vi "Set Value U64.vi"(0 "Session Handle in":T1, 1 "Create If Missing? (T)":bool=TRUE, 5 "Lookup String":string, 9 "Value":u64, 11 "error in (no error)":errorcluster) -> (4 "Session Handle out":T1, 15 "error out":errorcluster)   [LabVIEW 2019, in "HTS.lvlib" / "VariableContainer.lvclass"]
uses:
  VariableContainer.lvclass
  <vilib>/addons/TestStand/_TSUtility.llb/TestStand API Numeric Constants.ctl
  Typedefs/Session Handle.ctl
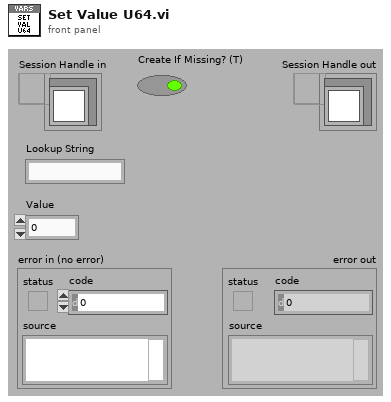
[diagram p1: front panel]
types:
  T1 = typedef "HTS.lvlib/VariableContainer.lvclass/Session Handle.ctl" = refnum<data-value>
  T2 = typedef "TestStand API Numeric Constants.ctl" = enum16{"APILocation_ActiveXModule_ActiveXReferenceExpr", "APILocation_ActiveXModule_FilePath", "APILocation_ActiveXModule_RemoteHost", "APILocation_ActiveXParameter_ValueExpr", "APILocation_AdditionalResult_Condition", "APILocation_AdditionalResult_Name", "APILocation_AdditionalResult_ValueToLog", "APILocation_CommonCModule_ModulePath", "APILocation_CommonCModule_ProjectFilePath", "APILocation_CommonCModule_SourceFilePath", "APILocation_CommonCModule_WorkspaceFilePath", "APILocation_CommonCParameter_StringBufferSizeExpr", "APILocation_CommonCParameter_ValueExpr", "APILocation_DllParameter_ImaginaryPartValueExpr", "APILocation_DotNetModule_GetAssembly", "APILocation_DotNetModule_ProjectFilePath", "APILocation_DotNetModule_SolutionFilePath", "APILocation_DotNetModule_SourceFilePath", "APILocation_DotNetParameter_ParameterName", "APILocation_DotNetParameter_ValueExpr", "APILocation_HTBasicModule_SubroutineFilePath", "APILocation_LabVIEWModule_CallName", "APILocation_LabVIEWModule_ClassPath", "APILocation_LabVIEWModule_GetVIAbsolutePath", "APILocation_LabVIEWModule_NodeLibraryName", "APILocation_LabVIEWModule_OverrideBinaryClassPath", "APILocation_LabVIEWModule_OverrideBinaryProjectPath", "APILocation_LabVIEWModule_OverrideBinaryVIPath", "APILocation_LabVIEWModule_OverrideSourceClassPath", "APILocation_LabVIEWModule_OverrideSourceProjectPath", "APILocation_LabVIEWModule_OverrideSourceVIPath", "APILocation_LabVIEWModule_ProjectPath", "APILocation_LabVIEWModule_RemoteConnectionTimeout", "APILocation_LabVIEWModule_RemoteHost", "APILocation_LabVIEWModule_RemotePortNumber", "APILocation_LabVIEWModule_VIPath", "APILocation_LabVIEWModule_VIType", "APILocation_LabVIEWNXGModule_GllPath", "APILocation_LabVIEWNXGModule_ModuleQualifiedName", "APILocation_LabVIEWNXGModule_ProjectPath", "APILocation_LabVIEWNXGModule_QualifiedName", "APILocation_LabVIEWNXGParameter_ParameterLabel", "APILocation_LabVIEWNXGParameter_Type", "APILocation_LabVIEWNXGParameter_ValueExpression", "APILocation_LabVIEWParameterElement_ElementCaption", "APILocation_LabVIEWParameterElement_ValueExpr", "APILocation_LabVIEWParameter_ParameterCaption", "APILocation_LabVIEWParameter_ValueExpr", "APILocation_None", "APILocation_PythonModule_ClassInstanceLocationExpr", "APILocation_PythonModule_ClassName", "APILocation_PythonModule_FunctionOrAttributeName", "APILocation_PythonModule_InterpreterReferenceExpr", "APILocation_PythonModule_ModulePath", "APILocation_PythonModule_PythonVersion", "APILocation_PythonModule_PythonVirtualEnvironmentPath", "APILocation_PythonParameter_ValueExpr", "APILocation_SequenceCallModule_CustomCPUAffinityForNewThread", "APILocation_SequenceCallModule_NewExecutionBreakOnEntryExpr", "APILocation_SequenceCallModule_NewExecutionModelPath", "APILocation_SequenceCallModule_NewExecutionTypeMaskExpr", "APILocation_SequenceCallModule_RemoteHost", "APILocation_SequenceCallModule_SequenceFilePath", "APILocation_SequenceCallModule_SequenceName", "APILocation_SequenceCallModule_StoreActiveXReferenceExpr", "APILocation_SequenceCallParameter_ValueExpr", "APILocation_SequenceFile_ModelPath", "APILocation_Sequence_DisableResults", "APILocation_StepType_BatchSyncOption", "APILocation_StepType_CustomActionExpression", "APILocation_StepType_CustomFalseAction", "APILocation_StepType_CustomFalseActionTargetByExpr", "APILocation_StepType_CustomTrueAction", "APILocation_StepType_CustomTrueActionTargetByExpr", "APILocation_StepType_DefaultNameExpr", "APILocation_StepType_DescriptionExpr", "APILocation_StepType_EvalPrecondForInteractiveExecution", "APILocation_StepType_FailAction", "APILocation_StepType_FailActionTargetByExpr", "APILocation_StepType_IconName", "APILocation_StepType_IgnoreRTE", "APILocation_StepType_LoopIncExpression", "APILocation_StepType_LoopInitExpression", "APILocation_StepType_LoopStatusExpression", "APILocation_StepType_LoopType", "APILocation_StepType_LoopWhileExpression", "APILocation_StepType_MenuItemNameExpr", "APILocation_StepType_ModuleLoadOption", "APILocation_StepType_ModuleUnloadOption", "APILocation_StepType_MutexNameOrRefExpr", "APILocation_StepType_PassAction", "APILocation_StepType_PassActionTargetByExpr", "APILocation_StepType_PostExpression", "APILocation_StepType_PreExpression", "APILocation_StepType_Precondition", "APILocation_StepType_RecordLoopIterationResults", "APILocation_StepType_RecordResult", "APILocation_StepType_ResultRecordingOption", "APILocation_StepType_RunMode", "APILocation_StepType_StatusExpression", "APILocation_StepType_StepFailCausesSequenceFail", "APILocation_StepType_SwitchExecConnectionLifetime", "APILocation_StepType_SwitchExecEnabled", "APILocation_StepType_SwitchExecMulticonnectMode", "APILocation_StepType_SwitchExecOperation", "APILocation_StepType_SwitchExecOperationOrder", "APILocation_StepType_SwitchExecRoutesToConnect", "APILocation_StepType_SwitchExecRoutesToDisconnect", "APILocation_StepType_SwitchExecVirtualDevice", "APILocation_StepType_SwitchExecWaitForDebounce", "APILocation_StepType_UseMutex", "APILocation_StepType_WindowActivation", "APILocation_Step_BatchSyncOption", "APILocation_Step_CustomActionExpression", "APILocation_Step_CustomFalseAction", "APILocation_Step_CustomFalseActionTargetByExpr", "APILocation_Step_CustomTrueAction", "APILocation_Step_CustomTrueActionTargetByExpr", "APILocation_Step_EvalPrecondForInteractiveExecution", "APILocation_Step_FailAction", "APILocation_Step_FailActionTargetByExpr", "APILocation_Step_IconName", "APILocation_Step_IgnoreRTE", "APILocation_Step_LoopIncExpression", "APILocation_Step_LoopInitExpression", "APILocation_Step_LoopStatusExpression", "APILocation_Step_LoopType", "APILocation_Step_LoopWhileExpression", "APILocation_Step_ModuleLoadOption", "APILocation_Step_ModuleUnloadOption", "APILocation_Step_MutexNameOrRefExpr", "APILocation_Step_PassAction", "APILocation_Step_PassActionTargetByExpr", "APILocation_Step_PostExpression", "APILocation_Step_PreExpression", "APILocation_Step_Precondition", "APILocation_Step_RecordLoopIterationResults", "APILocation_Step_RecordResult", "APILocation_Step_ResultRecordingOption", "APILocation_Step_RunMode", "APILocation_Step_StatusExpression", "APILocation_Step_StepFailCausesSequenceFail", "APILocation_Step_SwitchExecConnectionLifetime", "APILocation_Step_SwitchExecEnabled", "APILocation_Step_SwitchExecMulticonnectMode", "APILocation_Step_SwitchExecOperation", "APILocation_Step_SwitchExecOperationOrder", "APILocation_Step_SwitchExecRoutesToConnect", "APILocation_Step_SwitchExecRoutesToDisconnect", "APILocation_Step_SwitchExecVirtualDevice", "APILocation_Step_SwitchExecWaitForDebounce", "APILocation_Step_UniqueStepId", "APILocation_Step_UseMutex", "APILocation_Step_WindowActivation", "AcquireLicenseOption_NoOptions", "AcquireLicenseOption_ShowExitButton", "AcquireLicenseOption_SuppressStartupDialog", "AcquireLicenseOption_SuppressStartupDialogIfAlreadyShown", "AdditionalResultKind_Call", "AdditionalResultKind_Custom", "AdditionalResultKind_InParameter", "AdditionalResultKind_OutParameter", "AllowAutomaticTypeConflictResolutionOption_Always", "AllowAutomaticTypeConflictResolutionOption_Never", "AllowAutomaticTypeConflictResolutionOption_OnlyIfATypePaletteFileHasTheH", "AllowAutomaticTypeConflictResolutionOption_OnlyIfTypePaletteFilesWillNot", "ApplicationLicense_CustomEditor", "ApplicationLicense_OperatorInterface", "ApplicationLicense_SequenceEditor", "ApplicationLicense_Unspecified", "ApplicationSite_DefaultSite", "ApplicationSite_ItemList", "ApplicationSite_PropertyBrowser", "ApplicationSite_Settings", "ApplicationSite_Variables", "ArrayBounds_InitializeArray", "ArrayBounds_NoOptions", "ArrayBounds_ReturnOkCancel", "BatchSyncOption_NoSync", "BatchSyncOption_OneThreadOnly", "BatchSyncOption_Parallel", "BatchSyncOption_Serial", "BatchSyncOption_UseModelSetting", "BatchSyncOption_UseSeqFileSetting", "BlockFlag_AppliesToBlockStructure", "BlockFlag_Close", "BlockFlag_End", "BlockFlag_None", "BlockFlag_Open", "BlockFlag_Start", "BlockFlag_Unmatched", "BrowseExpr_ForViewingTypes", "BrowseExpr_ModalToAppMainWind", "BrowseExpr_NoContextMenus", "BrowseExpr_NoOptions", "BrowseExpr_UsesCRLF", "CPUAffinityForNewThreadOption_UseAffinityOfCaller", "CPUAffinityForNewThreadOption_UseAllCPUs", "CPUAffinityForNewThreadOption_UseCustomAffinity", "CPUAffinityForNewThreadOption_UseStationOption", "CallbackType_ModelPostError", "CallbackType_ModelPostFail", "CallbackType_ModelPostInteractive", "CallbackType_ModelPostResult", "CallbackType_ModelPostResults", "CallbackType_ModelPostStep", "CallbackType_ModelPreInteractive", "CallbackType_ModelPreStep", "CallbackType_SeqFilePostError", "CallbackType_SeqFilePostFail", "CallbackType_SeqFilePostInteractive", "CallbackType_SeqFilePostResult", "CallbackType_SeqFilePostResults", "CallbackType_SeqFilePostStep", "CallbackType_SeqFilePreInteractive", "CallbackType_SeqFilePreStep", "CallbackType_StationPostError", "CallbackType_StationPostFail", "CallbackType_StationPostInteractive", "CallbackType_StationPostResult", "CallbackType_StationPostResults", "CallbackType_StationPostStep", "CallbackType_StationPreInteractive", "CallbackType_StationPreStep", "CheckForModifiedTypes_AutoIncrementVersions", "CheckForModifiedTypes_NoAction", "CheckForModifiedTypes_Prompt", "CheckForModifiedTypes_RemoveTypesModifiedMark", "CheckForModifiedTypes_UseStationOptions", "CheckUpdatedStatusOption_All", "CheckUpdatedStatusOption_ExpectedGLLPath", "CheckUpdatedStatusOption_GVIChecksum", "CheckUpdatedStatusOption_GVIDescription", "CheckUpdatedStatusOption_GVIState", "CheckUpdatedStatusOption_QualifiedNamePresentInGLL", "CheckedState_Checked", "CheckedState_Indeterminate", "CheckedState_Unchecked", "CodeTemplateType_CVI", "CodeTemplateType_CppOrC", "CodeTemplateType_HTBasic", "CodeTemplateType_LabVIEW", "CodeTemplateType_LabVIEWNXG", "CodeTemplateType_Legacy", "CodeTemplateType_VisualBasicDotNet", "CodeTemplateType_VisualCSharpDotNet", "CodeTemplateType_VisualCppDotNet", "CommonDlgOption_ModalToAppMainWind", "CommonDlgOption_NoOptions", "CommonDlgOption_ReadOnly", "ConflictHandler_Error", "ConflictHandler_Prompt", "ConflictHandler_UseGlobalType", "CopyLocationsOption_DeepCopy", "CopyLocationsOption_ShallowCopy", "CrashCallbackOption_NoOptions", "CrashCallbackOption_PreloadFile", "CreateUndoItemOption_CreateOnly", "CreateUndoItemOption_NoOptions", "CustomUIMsgOptions_AppliesToAllThreads", "CustomUIMsgOptions_NoOptions", "CustomUIMsgOptions_SuppressIfTraceSent", "DebugOption_BufferChecking", "DebugOption_NoOptions", "DebugOption_ReportKnownOSandComponentProblems", "DebugOption_ReportObjectLeaks", "DebugOption_SendOutputMessagesToDebugger", "DebugOption_StackChecking", "DecimalPoint_UseComma", "DecimalPoint_UsePeriod", "DecimalPoint_UsePreference", "DecimalPoint_UseSystemSetting", "EditBreakAndWatch_DisplayBreakpointTab", "EditBreakAndWatch_DisplayWatchExpressionTab", "EditBreakAndWatch_ModalToAppMainWind", "EditBreakAndWatch_NoOptions", "EditBreakAndWatch_ReadOnly", "EditKind_ChangeNumericFormat", "EditKind_ChangeObject", "EditKind_ChangeRepresentation", "EditKind_ChangeRunMode", "EditKind_ChangeSequenceFileProperties", "EditKind_ChangeSequenceProperties", "EditKind_ChangeStep", "EditKind_ChangeValue", "EditKind_DeleteProperty", "EditKind_DeleteSequence", "EditKind_DeleteStep", "EditKind_InsertProperty", "EditKind_InsertSequence", "EditKind_InsertStep", "EditKind_InsertType", "EditKind_ModifyAttributes", "EditKind_ModifyComment", "EditKind_ModifyFlags", "EditKind_MoveProperty", "EditKind_MoveSequence", "EditKind_MoveStep", "EditKind_MoveType", "EditKind_None", "EditKind_Rename", "EditKind_ReplaceProperty", "EditNumFormat_AllowDefaultFormat", "EditNumFormat_ModalToAppMainWind", "EditNumFormat_NoOptions", "EditPaths_AllowEditOfReadOnlyFiles", "EditPaths_ModalToAppMainWind", "EditPaths_NoOptions", "EditPaths_ReadOnly", "EscapingOption_NoOptions", "EscapingOption_SurroundedByQuotes", "EvalOption_AllowEmptyExpression", "EvalOption_AllowIndexingEmptyArrays", "EvalOption_CreateNonExistentVariables", "EvalOption_DoNotAlterValues", "EvalOption_ForErrorChecking", "EvalOption_IgnoreNoValidationDirective", "EvalOption_NoOptions", "EvalPrecondOption_EvaluatePrecond", "EvalPrecondOption_NoEvaluatePrecond", "EvalPrecondOption_UseStationOption", "ExecMask_AllowBreakWhileInCodeModules", "ExecMask_BreakOnRunTimeError", "ExecMask_BreakWhileTerminating", "ExecMask_BreakpointsEnabled", "ExecMask_DefaultExecutionMask", "ExecMask_InteractiveEvaluatePreconditions", "ExecMask_InteractiveRecordResults", "ExecMask_InteractiveRunSetupCleanup", "ExecMask_TraceAllThreads", "ExecMask_TraceIntoEntryPoints", "ExecMask_TraceIntoPostActionCallbacks", "ExecMask_TraceIntoPrePostCallbacks", "ExecMask_TraceIntoSeparateExecutionCallbacks", "ExecMask_TraceIntoSequenceCallsMarkedAsTraceOff", "ExecMask_TraceIntoSetupCleanup", "ExecMask_TraceWhileTerminating", "ExecMask_TracingEnabled", "ExecRunState_Paused", "ExecRunState_Running", "ExecRunState_Stopped", "ExecTermState_Aborting", "ExecTermState_KillingThreads", "ExecTermState_Normal", "ExecTermState_Terminating", "ExecTermState_TerminatingInteractive", "ExecTypeMask_AutoWaitAtEndOfSequence", "ExecTypeMask_BreakOnSequenceFailure", "ExecTypeMask_BreakOnStepFailure", "ExecTypeMask_CloseWindowWhenDone", "ExecTypeMask_DiscardArgumentsWhenDone", "ExecTypeMask_DisplayPreloadProgress", "ExecTypeMask_InitiallyHidden", "ExecTypeMask_InitiallySuspended", "ExecTypeMask_Normal", "ExecTypeMask_NotRestartable", "ExecTypeMask_TracingInitiallyOff", "ExecTypeMask_UseSTA", "FailureAction_GotoCleanup", "FailureAction_None", "FailureAction_UseStationOption", "FileGlobalsScopeOption_AllExecutionsShare", "FileGlobalsScopeOption_SeparateForEachExecution", "FileModificationIndicatorPolicy_DefaultPolicy", "FileModificationIndicatorPolicy_ExcludeTestStandVersionUpgrade", "FileOpenMode_Append", "FileOpenMode_NoOptions", "FileOpenMode_Truncate", "FileOpenMode_Uniquify", "FileType_AdaptersConfigFile", "FileType_ConfigFile", "FileType_CustomConfigFile", "FileType_GeneralEngineConfigFile", "FileType_ProjectFile", "FileType_PropertyObjectFile", "FileType_SearchDirectoriesConfigFile", "FileType_SequenceFile", "FileType_StationGlobalsFile", "FileType_TemplatesFile", "FileType_TypePaletteFile", "FileType_TypePalettesConfigFile", "FileType_UsersFile", "FileType_WorkspaceFile", "FileVersionInc_Build", "FileVersionInc_Major", "FileVersionInc_Minor", "FileVersionInc_None", "FileVersionInc_Revision", "FileWritingFormat_Binary", "FileWritingFormat_Ini", "FileWritingFormat_Xml", "FindFile_AddDirToSrchList_Ask", "FindFile_AddDirToSrchList_Ask_IgnorePrivileges", "FindFile_AddDirToSrchList_No", "FindFile_AddDirToSrchList_Yes", "FindFile_AddDirToSrchList_Yes_IgnorePrivileges", "FindFile_PromptDisable", "FindFile_PromptEnable", "FindFile_PromptHonorUserPreference", "FindPath_PathIsDir", "FindPath_PathIsFile", "FindPath_PathNotFound", "FindPath_PathNotValid", "GetModuleFromProjectOption_NoOptions", "GetModuleFromProjectOption_NoPrompts", "GetSeqFile_AllowTypeConflicts", "GetSeqFile_CheckModelOptions", "GetSeqFile_DoNotRunLoadCallback", "GetSeqFile_FindFile", "GetSeqFile_GetFileOnlyIfInCache", "GetSeqFile_NoOptions", "GetSeqFile_OperatorInterfaceFlags", "GetSeqFile_PreloadModules", "GetSeqFile_SearchCurrentDir", "GetSeqFile_UpdateFromDisk", "GetTemplatesFileOption_LoadIfNotLoaded", "GetTemplatesFileOption_NoOptions", "GetUpdatedStatusOption_ExpectedGLLPathChanged", "GetUpdatedStatusOption_GVIChecksumChanged", "GetUpdatedStatusOption_GVIDescriptionChanged", "GetUpdatedStatusOption_GVIStateChanged", "GetUpdatedStatusOption_None", "GetUpdatedStatusOption_QualifiedNamePresentInGLL", "GotoLocationOption_DoNotDisplayMessageIfLocationNotFound", "GotoLocationOption_NoOptions", "HierarchicalExecMask_DontRunSetupAndCleanup", "HierarchicalExecMask_IgnorePreconditions", "HierarchicalExecMask_RunRemainingSequence", "InteractiveBranchMode_AllowAll", "InteractiveBranchMode_GotoEnd", "InteractiveBranchMode_Ignore", "InteractiveBranchMode_None", "InteractiveBranchMode_RaiseRTE", "InternalOption_ApplicationManager", "InternalOption_AutomationAdapterUsesDispatchForDualInterfaces", "InternalOption_DisableFloatingWindowsForModalDialogs", "InternalOption_UpdateExternalEnvironments", "InternalOption_WarnOnAPICallThroughDispatchInterface", "InternalStartupOption_TestStandReserved1", "LicenseType_BaseDeploymentEngine", "LicenseType_CustomEditorDeployment", "LicenseType_DebugDeploymentEnv", "LicenseType_DevelopmentSystem", "LicenseType_Evaluation", "LicenseType_NoLicense", "LicenseType_OEM", "LicenseType_Other", "LicenseType_Temporary", "LoadModule_DoNotPromptToFindFile", "LoadModule_DoNotRunLoadCallbacks", "LoadModule_EvaluateExpressions", "LoadModule_IgnoreErrors", "LoadModule_IgnoreSkippedSteps", "LoadModule_LoadModulesInSubSequences", "LoadModule_NoOptions", "LoadModule_ThrowExceptionOnError", "LoadOption_DynamicLoad", "LoadOption_PreloadWhenExecuted", "LoadOption_PreloadWhenOpened", "LoadOption_UseStepLoadOption", "LoadPrototypeOption_MapExistingParameters", "LoadPrototypeOption_NoOptions", "LoadTypePaletteOptions_DisplayErrors", "LoadTypePaletteOptions_NoOptions", "LocationKind_Execution", "LocationKind_File", "LocationKind_Type", "LockUnlockDialogOption_HideRememberPasswordControls", "LockUnlockDialogOption_Lock", "LockUnlockDialogOption_ModalToAppMainWind", "LockUnlockDialogOption_None", "LockUnlockDialogOption_Unlock", "ModelOption_NoModel", "ModelOption_RequireSpecificModel", "ModelOption_UseStationModel", "MsgBox_Custom", "MsgBox_Error", "MsgBox_Information", "MsgBox_Warning", "NewThreadOption_AutoWaitAtEndOfSequence", "NewThreadOption_InitiallySuspended", "NewThreadOption_NoOptions", "NewThreadOption_UseSTA", "OpenFile_DisableUseAbsPathCheck", "OpenFile_FileMustNotExist", "OpenFile_HideMultiSelectListCtrl", "OpenFile_HideUseAbsPathCheck", "OpenFile_IgnoreInitialPathExtension", "OpenFile_InitialSetBrowseIntoLLB", "OpenFile_InitialSetUseAbsPathCheck", "OpenFile_InitialUnsetUseAbsPathCheck", "OpenFile_ModalToAppMainWind", "OpenFile_NoOptions", "OpenFile_ResolveNonExistentFile", "OpenFile_SaveAsDialog", "OpenFile_SelectDirectoriesOnly", "OpenFile_ShowBrowseIntoLLBCheck", "OpenFile_SubstituteMacrosByDefault", "OpenFile_UseAbsolutePath", "OpenFile_UseRelativePath", "OpenFile_UseSequenceFileFilters", "OpenStatus_InWindow", "OpenWorkspaceFile_IgnoreMissingFiles", "OpenWorkspaceFile_NoOptions", "OpenWorkspaceFile_SearchCurrentDirectory", "OpenWorkspaceFile_UseSearchDirectories", "OutputMessageSeverity_Error", "OutputMessageSeverity_Information", "OutputMessageSeverity_Warning", "ParseLookupStringOption_NoOptions", "ParseLookupStringOption_TreatArrayIndicesAsSeparateTokens", "PerformActionOption_No", "PerformActionOption_Prompt", "PerformActionOption_Yes", "PostResultsCallbackMaskOption_All", "PostResultsCallbackMaskOption_None", "PostResultsCallbackMaskOption_PostAction", "PostResultsCallbackMaskOption_PostInteractive", "PostResultsCallbackMaskOption_PostResultListEntry", "PostResultsCallbackMaskOption_PostStep", "PostResultsCallbackMaskOption_PostStepFailure", "PostResultsCallbackMaskOption_PostStepRuntimeError", "PostResultsCallbackMaskOption_PreInteractive", "PostResultsCallbackMaskOption_PreStep", "PostResultsCallbackMaskOption_SequenceCall", "PostResultsCallbackOption_CallAfterProvisionalResult", "PostResultsCallbackOption_NoOptions", "ProfilerOption_ExcludeLoad", "ProfilerOption_ExcludeLocationInformation", "ProfilerOption_ExcludeProcessModels", "ProfilerOption_ExcludeStepModules", "ProfilerOption_ExcludeStepTypeModules", "ProfilerOption_ExcludeSteps", "ProfilerOption_ExcludeSynchronization", "ProfilerOption_ExcludeUnload", "ProfilerOption_NoOptions", "ProfilerState_Aborted", "ProfilerState_Blocked", "ProfilerState_Completed", "ProfilerState_InUse", "ProfilerState_NotAState", "ProfilerState_TimedOut", "PromptResult_Cancel", "PromptResult_No", "PromptResult_Yes", "PropDlgOption_DisableAdvancedButton", "PropDlgOption_DisableNumericFormatButton", "PropDlgOption_ModalToAppMainWind", "PropDlgOption_NoOptions", "PropDlgOption_ReadOnly", "PropDlgOption_ShowViewContentsButton", "PropDlgOption_UseVariablesViewDialog", "PropDlgOutput_AppliedChanges", "PropDlgOutput_AppliedToAllInstances", "PropDlgOutput_ModifiedFile", "PropDlgOutput_ModifiedObject", "PropDlgOutput_ViewContents", "PropFlags_CommentNotEditable", "PropFlags_DontCopyToResults", "PropFlags_DontTypeCheckParameter", "PropFlags_ExcludeFromComparison", "PropFlags_ExcludeFromCopy", "PropFlags_Hidden", "PropFlags_HiddenInTypes", "PropFlags_IncludeInReport", "PropFlags_IntermediateExprValue", "PropFlags_IsLimit", "PropFlags_IsMeasurementValue", "PropFlags_NameNotEditable", "PropFlags_NotDeletable", "PropFlags_NotEditable", "PropFlags_PassByReference", "PropFlags_PermitPropagation", "PropFlags_Propagate", "PropFlags_SerializeAlias", "PropFlags_Shared", "PropFlags_SharedAtRunTime", "PropFlags_UnstructuredProperty", "PropOption_CaseInsensitive", "PropOption_Coerce", "PropOption_CoerceBadNumbersToZero", "PropOption_CoerceFromBoolean", "PropOption_CoerceFromEnum", "PropOption_CoerceFromNumber", "PropOption_CoerceFromReference", "PropOption_CoerceFromString", "PropOption_CoerceToBoolean", "PropOption_CoerceToEnum", "PropOption_CoerceToNumber", "PropOption_CoerceToReference", "PropOption_CoerceToString", "PropOption_CopyAllFlags", "PropOption_DecimalPoint_UseComma", "PropOption_DecimalPoint_UsePeriod", "PropOption_DecimalPoint_UsePreference", "PropOption_DecimalPoint_UseSystemSetting", "PropOption_DeleteIfExists", "PropOption_DoNotAdoptCurrentName", "PropOption_DoNotRecurse", "PropOption_DoNotShareProperties", "PropOption_DoNothingIfExists", "PropOption_InsertElement", "PropOption_InsertIfMissing", "PropOption_NoOptions", "PropOption_NotOwning", "PropOption_OverrideNotDeletable", "PropOption_ReferToAlias", "PropOption_RemoveElement", "PropOption_RequireIdenticalStructure", "PropOption_SetOnlyIfDoesNotExist", "PropTypeFlags_DisableEditingInstanceFlags", "PropTypeFlags_IsModifiedType", "PropTypeFlags_NIInstalledType", "PropTypeFlags_NoAutoConvertVersions", "PropTypeFlags_NoFlags", "PropTypeFlags_PreventEditingType", "PropValTypeFlag_Any", "PropValTypeFlag_ArrayOfNamedType", "PropValTypeFlag_Boolean", "PropValTypeFlag_BooleanArray", "PropValTypeFlag_Container", "PropValTypeFlag_ContainerArray", "PropValTypeFlag_Enum", "PropValTypeFlag_NamedType", "PropValTypeFlag_Nothing", "PropValTypeFlag_Number", "PropValTypeFlag_NumberArray", "PropValTypeFlag_Object", "PropValTypeFlag_PlainContainer", "PropValTypeFlag_PlainReference", "PropValTypeFlag_Reference", "PropValTypeFlag_ReferenceArray", "PropValTypeFlag_String", "PropValTypeFlag_StringArray", "PropValType_Array", "PropValType_Boolean", "PropValType_Container", "PropValType_Enum", "PropValType_NamedType", "PropValType_Number", "PropValType_Reference", "PropValType_String", "PropertyObjectElement_Attributes", "PropertyObjectElement_Comment", "PropertyObjectElement_Flags", "PropertyObjectElement_Name", "PropertyObjectElement_None", "PropertyObjectElement_NumericFormat", "PropertyObjectElement_Representation", "PropertyObjectElement_Value", "PropertyRepresentation_Float64", "PropertyRepresentation_Int64", "PropertyRepresentation_None", "PropertyRepresentation_UInt64", "ProtectedObjectOption_None", "ProtectedObjectOption_NotEditable", "ProtectedObjectOption_NotViewable", "RTEOption_Abort", "RTEOption_Continue", "RTEOption_Ignore", "RTEOption_Retry", "RTEOption_ShowDialog", "RWOption_DoNotWriteTypes", "RWOption_EraseAll", "RWOption_EraseExistingObject", "RWOption_NoOptions", "RWOption_ValuesOnly", "ReadPropertyObjectFileOption_None", "ReadPropertyObjectFileOption_TypesOnly", "ReleaseSeqFile_DoNotRunUnloadCallback", "ReleaseSeqFile_NoOptions", "ReleaseSeqFile_UnloadFile", "ReleaseSeqFile_UnloadFileIfModified", "ReportConv_FromCRLF", "ReportConv_NoConversion", "ReportConv_ToCRLF", "ResetTypeInst_NoOptions", "ResetTypeInst_RecurseSubProperties", "ResetTypeInst_ResetFlags", "ResetTypeInst_ResetValues", "RestartOption_BreakOnEntry", "RestartOption_BreakOnSequenceFailure", "RestartOption_BreakOnStepFailure", "RestartOption_NoOptions", "RestartOption_OverrideNotRestartable", "ResultLogRecordType_BatchDone", "ResultLogRecordType_BatchStart", "ResultLogRecordType_Begin", "ResultLogRecordType_Deleted", "ResultLogRecordType_End", "ResultLogRecordType_NotARecordType", "ResultLogRecordType_OnTheFlyStepResults", "ResultLogRecordType_PostBatch", "ResultLogRecordType_PostUUT", "ResultLogRecordType_PreBatch", "ResultLogRecordType_PreUUT", "ResultLogRecordType_UUTDone", "ResultLogRecordType_UUTStart", "ResultRecordingOption_Disabled", "ResultRecordingOption_Enabled", "ResultRecordingOption_EnabledAndOverrideSequenceSetting", "SCCmdOption_DoNotRecurse", "SCCmdOption_NoOptions", "SCCmdOption_ShowPromptDialog", "SCCmdOption_SkipErrorDialog", "SCCmdOption_SkipPromptDialog", "SCCmd_AddToSC", "SCCmd_CheckIn", "SCCmd_CheckOut", "SCCmd_GetLatest", "SCCmd_RemoveFromSC", "SCCmd_ShowDifferences", "SCCmd_ShowHistory", "SCCmd_ShowProperties", "SCCmd_ShowProviderOptions", "SCCmd_UndoCheckOut", "SCStatus_CheckedOut", "SCStatus_CheckedOutByUser", "SCStatus_CheckedOutMultiple", "SCStatus_CheckedOutOther", "SCStatus_Deleted", "SCStatus_InSC", "SCStatus_NotInSC", "SCStatus_OutOfDate", "SaveAllSeqFiles_NoOptions", "SaveAllSeqFiles_PromptUser", "SaveWorkspaceFile_NoOptions", "SaveWorkspaceFile_PromptUser", "SaveWorkspaceFile_SkipReadOnlyFiles", "SaveWorkspaceFile_SkipWorkspaceFile", "SearchDirectoryType_AdapterSupportDir", "SearchDirectoryType_ApplicationDir", "SearchDirectoryType_ContainingProjectDir", "SearchDirectoryType_CurrentSequenceFileDir", "SearchDirectoryType_CurrentWorkspaceDir", "SearchDirectoryType_ExplicitDir", "SearchDirectoryType_InitialWorkingDir", "SearchDirectoryType_NIComponentsDir", "SearchDirectoryType_PathEnvironmentVarDir", "SearchDirectoryType_PublicComponentsDir", "SearchDirectoryType_TestStandBinDir", "SearchDirectoryType_TestStandDir", "SearchDirectoryType_TestStandPublicDir", "SearchDirectoryType_UserComponentsDir", "SearchDirectoryType_WindowsDir", "SearchDirectoryType_WindowsSystemDir", "SearchElement_All", "SearchElement_AllValues", "SearchElement_Attributes", "SearchElement_BooleanValue", "SearchElement_Comment", "SearchElement_Enumerators", "SearchElement_Name", "SearchElement_NumericValue", "SearchElement_StringValue", "SearchElement_TypeName", "SearchFilterOptions_All", "SearchFilterOptions_BuiltinSeqAndSeqFileProps", "SearchFilterOptions_BuiltinStepProps", "SearchFilterOptions_CustomDataTypes", "SearchFilterOptions_CustomStepProps", "SearchFilterOptions_FileGlobals", "SearchFilterOptions_Locals", "SearchFilterOptions_ModuleStepProps", "SearchFilterOptions_Parameters", "SearchFilterOptions_StandardDataTypes", "SearchFilterOptions_StepTypes", "SearchFilterOptions_Steps", "SearchFilterOptions_TypesOnly", "SearchOptions_IncludeSubsequenceFiles", "SearchOptions_MatchCase", "SearchOptions_RegExpr", "SearchOptions_WholeWordOnly", "SeqDefValueScope_Execution", "SeqDefValueScope_ExecutionTree", "SeqFileBatchSyncOption_NoSync", "SeqFileBatchSyncOption_OneThreadOnly", "SeqFileBatchSyncOption_Parallel", "SeqFileBatchSyncOption_Serial", "SeqFileBatchSyncOption_UseModelSetting", "SeqFileType_FrontEndCBacks", "SeqFileType_Model", "SeqFileType_Normal", "SeqFileType_StationCBacks", "SeqFileType_Template", "SeqType_Callback", "SeqType_CfgEntryPoint", "SeqType_ExeEntryPoint", "SeqType_Normal", "SeqType_ReservedCallback", "SequenceFileDifferOptions_IgnoreUniqueStepId", "SequenceFileDifferOptions_NoOptions", "SequenceFileDifferenceType_ArrayDimensions", "SequenceFileDifferenceType_Attributes", "SequenceFileDifferenceType_ChangeComment", "SequenceFileDifferenceType_ChangeFlags", "SequenceFileDifferenceType_ChangeNumericFormat", "SequenceFileDifferenceType_ChangeType", "SequenceFileDifferenceType_ChangeValue", "SequenceFileDifferenceType_Delete", "SequenceFileDifferenceType_Insert", "SequenceFileDifferenceType_NoDifference", "SequenceFileDifferenceType_SubProperties", "SequenceFileDifferenceType_UnknownProblem", "SerializationOption_NoOptions", "SerializationOption_SupportNonTypedefMatchingInstances", "SerializationOption_UseBinary", "SerializationOption_UseXml", "SetTempFileDirectoryOption_Default", "SetTempFileDirectoryOption_NeverOverride", "SpecMod_AllowPrototypeChanges", "SpecMod_NoOptions", "SpecMod_NoParameterLogging", "SpecMod_NoSyntaxChecking", "SpecMod_ReadOnly", "SpecifyStepsByUniqueIdOption_Ask", "SpecifyStepsByUniqueIdOption_No", "SpecifyStepsByUniqueIdOption_Yes", "StepDescOption_IncludeBreakpoint", "StepDescOption_Long", "StepDescOption_NoOptions", "StepGroup_Cleanup", "StepGroup_Main", "StepGroup_Setup", "SwitchExecLifetime_Execution", "SwitchExecLifetime_Manual", "SwitchExecLifetime_Sequence", "SwitchExecLifetime_Step", "SwitchExecLifetime_Thread", "SwitchExecMulticonnectMode_Default", "SwitchExecMulticonnectMode_Multiconnect", "SwitchExecMulticonnectMode_None", "SwitchExecOperationOrder_DisconnectAfterConnect", "SwitchExecOperationOrder_DisconnectBeforeConnect", "SwitchExecOperation_Connect", "SwitchExecOperation_ConnectDisconnect", "SwitchExecOperation_Disconnect", "SwitchExecOperation_DisconnectAll", "TS_Err_AccessDenied", "TS_Err_ActiveXAutomationServerException", "TS_Err_AdapterNoConnectToAutoServer", "TS_Err_AdapterServerConnectionLost", "TS_Err_ArrayDimensionExpected", "TS_Err_ArrayDimensionSizeExpected", "TS_Err_ArrayIndexOutOfBounds", "TS_Err_ArrayLocked", "TS_Err_ArrayTypeExpected", "TS_Err_AutomationObjNotValid", "TS_Err_BadExpressionError", "TS_Err_BadFileFormat", "TS_Err_BadNetPath", "TS_Err_BadPropertyOrVariableName", "TS_Err_CVIAutoCmdFailed", "TS_Err_CVICantConnectToTecrunServer", "TS_Err_CVIFuncNotFoundInModule", "TS_Err_CVIModuleHasUnresolvedReferences", "TS_Err_CVINonDllModuleNotSupported", "TS_Err_CVINotReg", "TS_Err_CVIOleError", "TS_Err_CVIRegGenericReadError", "TS_Err_CVIRegKeyNotFound", "TS_Err_CVIRegValueNotFound", "TS_Err_CVIRegValueTypeMismatch", "TS_Err_CVIUnableToTerminateUserProgInCVI", "TS_Err_CVIVersionNotSupported", "TS_Err_ConvertedErrorCode", "TS_Err_CurrentSeqFileNotAvailable", "TS_Err_DDEFail", "TS_Err_DLLNotLoadable", "TS_Err_DNAssemblyMissing", "TS_Err_DiskFull", "TS_Err_DispMissingParamID", "TS_Err_DispMissingParamName", "TS_Err_DispMissingRequiredArg", "TS_Err_DispObsoleteMember", "TS_Err_DispUnknownInterface", "TS_Err_DispUnknownMemberID", "TS_Err_DispUnknownMemberName", "TS_Err_DispUnknownParamID", "TS_Err_DispUnknownParamName", "TS_Err_DispWrongNumPositionalParams", "TS_Err_DoesNotHaveRequiredPrivilege", "TS_Err_DriveNotReady", "TS_Err_DuplicateItemOrValue", "TS_Err_EmptyExpressionError", "TS_Err_EvaluateFunctionEmptyExpressionError", "TS_Err_EvaluationContextNotAvailable", "TS_Err_ExprTypeIncompatibleWithParameter", "TS_Err_ExprValueNotSuperSetOfParameter", "TS_Err_ExternalServerUnavailable", "TS_Err_FailToRegisterClipFormat", "TS_Err_FileAlreadyExists", "TS_Err_FileFormatIsOutOfDate", "TS_Err_FileFormatNewerThanCurrentVersion", "TS_Err_FileNotConvertableToSeqFile", "TS_Err_FileWasNotFound", "TS_Err_FunctionNotFoundInLib", "TS_Err_IOError", "TS_Err_IllegalOperationOnValue", "TS_Err_IncompatibleParameters", "TS_Err_IndexOutOfRange", "TS_Err_Int32Overflow", "TS_Err_Int64Overflow", "TS_Err_InvalidAdapterName", "TS_Err_InvalidDrive", "TS_Err_InvalidPathname", "TS_Err_InvalidPointer", "TS_Err_InvalidRegularExpression", "TS_Err_ItemCannotBeDeleted", "TS_Err_LVAutoServerError", "TS_Err_LVMissingRequiredArg", "TS_Err_LVRTDllNotLoaded", "TS_Err_LVReportedError", "TS_Err_LVRunTimeEngineError", "TS_Err_LVTypeConversionError", "TS_Err_LV_NXG_AutoBuildError", "TS_Err_LV_NXG_AutoServerError", "TS_Err_LV_NXG_MissingRequiredArg", "TS_Err_LV_NXG_RTEDllNotLoaded", "TS_Err_LV_NXG_ReportedError", "TS_Err_LV_NXG_RunTimeEngineError", "TS_Err_LV_NXG_TypeConversionError", "TS_Err_LValueExpected", "TS_Err_LabVIEWTypeNotSupportedInCVI", "TS_Err_MeasStudioInterfaceNotFound", "TS_Err_MemoryChecking", "TS_Err_MethodOrPropertyNotAvailable", "TS_Err_MismatchedArrayBounds", "TS_Err_MismatchedItems", "TS_Err_MissingType", "TS_Err_ModuleLoadFailure", "TS_Err_ModuleNotSpecified", "TS_Err_NameAlreadyInUse", "TS_Err_NoError", "TS_Err_NoFileAssoc", "TS_Err_NoItemsInList", "TS_Err_NotSupported", "TS_Err_OS_Exception", "TS_Err_ObjectCannotBeAdded", "TS_Err_ObjectLocked", "TS_Err_ObjectTypeIncompatibleWithParameter", "TS_Err_OperationCanceled", "TS_Err_OperationFailed", "TS_Err_OperationInProgress", "TS_Err_OperationOnlyValidWhenSuspended", "TS_Err_OperationTimedOut", "TS_Err_OutOfMemory", "TS_Err_PathNotFound", "TS_Err_ProgramError", "TS_Err_RStringNotFound", "TS_Err_ReadObjectNotFound", "TS_Err_RegistryAccessError", "TS_Err_RegistryItemNotFound", "TS_Err_RemoteHostNotSpecified", "TS_Err_RemoteSequenceError", "TS_Err_RemoteSequenceErrorUnableToConnect", "TS_Err_RemoteSequenceRemoteExecutionDenied", "TS_Err_SequenceAborted", "TS_Err_SequenceTerminated", "TS_Err_SharingViolation", "TS_Err_SingleDimensionalNumericArrayExpected", "TS_Err_SourceCodeControlError", "TS_Err_StackOverflow", "TS_Err_StepTypeNotFound", "TS_Err_ThreadCreationFailed", "TS_Err_TooManyItems", "TS_Err_TwoDimensionalNumericArrayExpected", "TS_Err_TypeCannotBeDeleted", "TS_Err_TypeConflict", "TS_Err_TypeLibraryReadError", "TS_Err_TypeMismatchError", "TS_Err_TypePaletteFileLoadErrors", "TS_Err_TypeWithDependingInstancesCannotBeDeleted", "TS_Err_UInt32Overflow", "TS_Err_UInt64Overflow", "TS_Err_UnRecognizedValue", "TS_Err_UnableToAllocateSystemResource", "TS_Err_UnableToCloseFile", "TS_Err_UnableToInitializeOLESystemDLLs", "TS_Err_UnableToLaunchCVI", "TS_Err_UnableToOpenDirectory", "TS_Err_UnableToOpenFile", "TS_Err_UnableToPassByReference", "TS_Err_UnexpectedChangeCount", "TS_Err_UnexpectedEndOfFile", "TS_Err_UnexpectedSystemError", "TS_Err_UnexpectedType", "TS_Err_UnknownFunctionOrSequenceName", "TS_Err_UnknownType", "TS_Err_UnknownVariableOrProperty", "TS_Err_ValueIsInvalidOrOutOfRange", "TS_Err_VisualStudioAutomationError", "TS_Err_WatchExpressionError", "TS_Err_WriteProtected", "TS_Err_WrongNumberOfArrayIndices", "TS_Err_WrongNumberOfParameters", "TS_Err_XMLError", "TestStandPath_Bin", "TestStandPath_CommonAppData", "TestStandPath_Config", "TestStandPath_GlobalCommonAppData", "TestStandPath_GlobalConfig", "TestStandPath_GlobalLocalAppData", "TestStandPath_GlobalPublic", "TestStandPath_LocalAppData", "TestStandPath_NIComponents", "TestStandPath_Public", "TestStandPath_PublicComponents", "TestStandPath_Temp", "TestStandPath_Temporary", "TestStandPath_TestStand", "ThreadTerminationOption_Never", "ThreadTerminationOption_Normal", "ThreadTerminationOption_Prompt", "TimeLimitAction_Abort", "TimeLimitAction_KillThreads", "TimeLimitAction_Prompt", "TimeLimitAction_Terminate", "TimeLimitOperation_Aborting", "TimeLimitOperation_Executing", "TimeLimitOperation_Terminating", "TimeLimitType_Exiting", "TimeLimitType_NormalExecution", "TokenCode_Assignment", "TokenCode_Bad", "TokenCode_BinaryInteger", "TokenCode_BitwiseAnd", "TokenCode_BitwiseAndAssignment", "TokenCode_BitwiseNot", "TokenCode_BitwiseOr", "TokenCode_BitwiseOrAssignment", "TokenCode_Colon", "TokenCode_Conditional", "TokenCode_Directive", "TokenCode_DivAssignment", "TokenCode_Divide", "TokenCode_DotDot", "TokenCode_Equal", "TokenCode_ExclusiveOr", "TokenCode_ExclusiveOrAssignment", "TokenCode_FieldSpecifier", "TokenCode_GreaterThan", "TokenCode_GreaterThanEqual", "TokenCode_HexInteger", "TokenCode_Identifier", "TokenCode_Integer", "TokenCode_Integer64", "TokenCode_LeftBrace", "TokenCode_LeftBracket", "TokenCode_LeftParenthesis", "TokenCode_LeftShift", "TokenCode_LeftShiftAssignment", "TokenCode_LessThan", "TokenCode_LessThanEqual", "TokenCode_LogicalAnd", "TokenCode_LogicalNot", "TokenCode_LogicalOr", "TokenCode_Minus", "TokenCode_MinusAssignment", "TokenCode_MinusMinus", "TokenCode_ModAssignment", "TokenCode_Modulus", "TokenCode_MultAssignment", "TokenCode_MultiLineComment", "TokenCode_Multiply", "TokenCode_NotAToken", "TokenCode_NotEqual", "TokenCode_OctalInteger", "TokenCode_Plus", "TokenCode_PlusAssignment", "TokenCode_PlusPlus", "TokenCode_Real", "TokenCode_ReferenceFieldSpecifier", "TokenCode_RightBrace", "TokenCode_RightBracket", "TokenCode_RightParenthesis", "TokenCode_RightShift", "TokenCode_RightShiftAssignment", "TokenCode_Separator", "TokenCode_SingleLineComment", "TokenCode_String", "TokenCode_SymbolicConstant", "TokenCode_UnescapedString", "TokenCode_UnsignedInteger64", "TokenCode_UnterminatedMultiLineComment", "TokenCode_UnterminatedString", "TokenizeOption_NoOptions", "TokenizeOption_PreserveComments", "TokenizeOption_RecognizeCPPIdentifiers", "TokenizeOption_RecognizeIncompleteExpression", "ToolMenuItem_EditsSelectedFile", "ToolMenuItem_Enabled", "ToolMenuItem_SeparatorBefore", "ToolMenuType_Command", "ToolMenuType_Sequence", "ToolMenuType_SequenceFile", "ToolMenuType_SubMenu", "TypeCategory_BuiltinDataTypes", "TypeCategory_CustomDataTypes", "TypeCategory_None", "TypeCategory_StepTypes", "TypeEqualOption_DoNotCompareDimensions", "TypeEqualOption_DoNotCompareIsObject", "TypeEqualOption_NoOptions", "TypeVersionInc_Build", "TypeVersionInc_Major", "TypeVersionInc_Minor", "TypeVersionInc_None", "TypeVersionInc_Revision", "UIMsg_AbortingExecution", "UIMsg_BreakOnBreakpoint", "UIMsg_BreakOnRunTimeError", "UIMsg_BreakOnUserRequest", "UIMsg_CascadeWindows", "UIMsg_ClientFileChanged", "UIMsg_CloseWindows", "UIMsg_DisplayReport", "UIMsg_EndExecution", "UIMsg_EndFileExecution", "UIMsg_EndInteractiveExecution", "UIMsg_GotoLocation", "UIMsg_KillingExecutionThreads", "UIMsg_LocalizationSettingChanged", "UIMsg_ModelState_BeginTesting", "UIMsg_ModelState_EnabledStateSet", "UIMsg_ModelState_Identified", "UIMsg_ModelState_Initializing", "UIMsg_ModelState_PostProcessing", "UIMsg_ModelState_PostProcessingComplete", "UIMsg_ModelState_TestingComplete", "UIMsg_ModelState_Waiting", "UIMsg_NonTerminatableThreadsArePreventingTermination", "UIMsg_OpenWindows", "UIMsg_OutputMessages", "UIMsg_ProgressPercent", "UIMsg_ProgressText", "UIMsg_PushUndoItem", "UIMsg_RefreshWindows", "UIMsg_ReportChanged", "UIMsg_ReportCollectionChanged", "UIMsg_ReportLocationChanged", "UIMsg_ResumeFromBreak", "UIMsg_RuntimeError", "UIMsg_ShutDownCancelled", "UIMsg_ShutDownComplete", "UIMsg_StartExecution", "UIMsg_StartFileExecution", "UIMsg_StartInteractiveExecution", "UIMsg_TerminatingExecution", "UIMsg_TerminatingInteractiveExecution", "UIMsg_TerminationCancelled", "UIMsg_TileWindows", "UIMsg_Trace", "UIMsg_TypePaletteFileListChanged", "UIMsg_UserMessageBase", "UnloadOption_AfterSequenceExecution", "UnloadOption_AfterStepExecution", "UnloadOption_OnPreconditionFailure", "UnloadOption_UseStepUnloadOption", "UnloadOption_WithSequenceFile", "UpdateModuleFromStepOption_CopyParameterDefaultCheckState", "UpdateModuleFromStepOption_CopyParameterLogCheckState", "UpdateModuleFromStepOption_CopyParameterValue", "UpdateModuleFromStepOption_CopyShowFrontPanelState", "UpdateModuleFromStepOption_CopyStepRTEState", "UpdateModuleFromStepOption_None", "ValidateOverrideSettingsOption_All", "ValidateOverrideSettingsOption_OverrideBinaryClassPath", "ValidateOverrideSettingsOption_OverrideBinaryProjectPath", "ValidateOverrideSettingsOption_OverrideBinaryVIPath", "ValidateOverrideSettingsOption_OverrideClassPath", "ValidateOverrideSettingsOption_OverrideProjectPath", "ValidateOverrideSettingsOption_OverrideVIPath", "ValidateOverrideSettingsOption_VIPPLInSync", "VersionConstant_BuildVersion", "VersionConstant_MajorVersion", "VersionConstant_MinorVersion", "VersionConstant_RevisionVersion", "WatchExpressionBreakType_None", "WatchExpressionBreakType_OnChange", "WatchExpressionBreakType_OnExpressionTrue", "WatchExpressionFilter_FilterByExecution", "WatchExpressionFilter_FilterBySequence", "WatchExpressionFilter_FilterBySequenceFile", "WatchExpressionFilter_IncludeGlobals", "WatchExpressionFilter_NoOptions", "WinActOption_ActivateWhenStepCompletes", "WinActOption_IfActiveReactivateWhenStepCompletes", "WinActOption_None", "WinFileDlg_ALLOWMULTISELECT", "WinFileDlg_CREATEPROMPT", "WinFileDlg_DONTADDTORECENT", "WinFileDlg_ENABLEHOOK", "WinFileDlg_ENABLEINCLUDENOTIFY", "WinFileDlg_ENABLESIZING", "WinFileDlg_ENABLETEMPLATE", "WinFileDlg_ENABLETEMPLATEHANDLE", "WinFileDlg_EXPLORER", "WinFileDlg_EXTENSIONDIFFERENT", "WinFileDlg_FILEMUSTEXIST", "WinFileDlg_FORCESHOWHIDDEN", "WinFileDlg_HIDEREADONLY", "WinFileDlg_LONGNAMES", "WinFileDlg_NOCHANGEDIR", "WinFileDlg_NODEREFERENCELINKS", "WinFileDlg_NOLONGNAMES", "WinFileDlg_NONETWORKBUTTON", "WinFileDlg_NOREADONLYRETURN", "WinFileDlg_NOTESTFILECREATE", "WinFileDlg_NOVALIDATE", "WinFileDlg_OVERWRITEPROMPT", "WinFileDlg_PATHMUSTEXIST", "WinFileDlg_READONLY", "WinFileDlg_SHAREAWARE", "WinFileDlg_SHOWHELP", "WorkspaceBrowserDlgOption_Editable", "WorkspaceBrowserDlgOption_ModalToAppMainWind", "WorkspaceBrowserDlgOption_NoOptions", "WorkspaceObjType_Folder", "WorkspaceObjType_OtherFile", "WorkspaceObjType_ProjectFile", "WorkspaceObjType_SequenceFile", "WorkspaceObjType_WorkspaceFile", "WriteFileFormat_Current", "WriteFileFormat_TestStand3", "WriteFileFormat_TestStand31", "WriteFileFormat_TestStand35", "WriteFileFormat_TestStand4", "WriteFileFormat_TestStand41", "WriteFileFormat_TestStand42", "WriteFileFormat_TestStand45", "WriteFileFormat_TestStand50", "WriteFileFormat_TestStand51", "WriteFileFormat_TestStand_14_0", "WriteFileFormat_TestStand_16_0", "WriteFileFormat_TestStand_17", "WriteFileFormat_TestStand_19", "XMLOption_AllowInvalidObjects", "XMLOption_ExcludeAliasObjects", "XMLOption_ExcludeArrayPrototypes", "XMLOption_ExcludeAttributes", "XMLOption_ExcludeComments", "XMLOption_ExcludeEmptyObjects", "XMLOption_ExcludeFlags", "XMLOption_ExcludeVersionInfo", "XMLOption_NoCRLF", "XMLOption_NoIndentation", "XMLOption_NoOptions", "XMLOption_UseCRLFInsteadOfLF", "XMLOption_UseValueFormatIfDefined"}
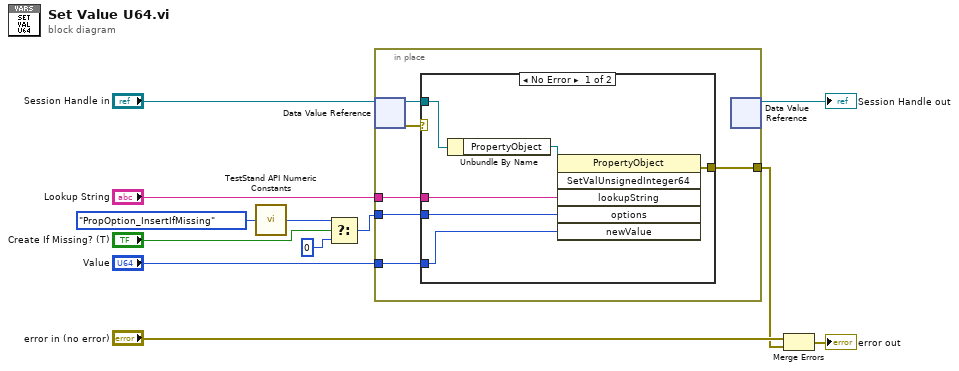
[diagram p0: block diagram]
diagram:
  n1 = call <vilib>:"TestStand API Numeric Constants.vi"("Constant"=TestStand_API_Numeric_Constants."PropOption_InsertIfMissing") -> ("Value"=w9:i32)  [unwired: 4 out]
  n2 = Select(t=w9, s="Create If Missing? (T)", f=0) -> (s? t:f=w3:i32)
  n3 = in-place {
    in-place-border: "Lookup String" -> [w17]
    in-place-border: [w15] -> w4
    in-place-border: w3 -> [w14]
    in-place-border: "Value" -> [w13]
    n4 = in-place-dvr #1("Session Handle in") -> (w18:refnum<class "VariableContainer.lvclass">, w16:errorcluster)
    n5 = case shown="No Error" w16 {
      selector: w16 -> [_ w25]
      tunnel: w18 -> [w24 _]
      tunnel: w17 -> [w22 _]
      tunnel: [w21 w25] -> w15
      tunnel: w14 -> [w20 _]
      tunnel: w13 -> [w19 _]
      frame No Error {
        n6 = Unbundle By Name(w24) -> ("PropertyObject"=w23:refnum<k7>)
        n7 = invoke class="PropertyObject" method="SetValUnsignedInteger64"(reference=w23, "lookupString"=w22, "options"=w20, "newValue"=w19) -> (error out=w21:errorcluster)  [unwired: 2 in, 5 out]
      }
      frame Error {
      }
    }
    n8 = in-place-dvr #1() -> (→"Session Handle out":T1)  [unwired: 1 in, 1 out]
  }
  n9 = Merge Errors("error in (no error)", w4) -> (→"error out":errorcluster)
